vi "Test CVT.vi"() -> ()   [LabVIEW 2014, in "Controller.lvlib" / "Controller.lvclass"]
uses:
  Controller.lvclass
panel:
  out "data value":variant
  out "json cvt":string
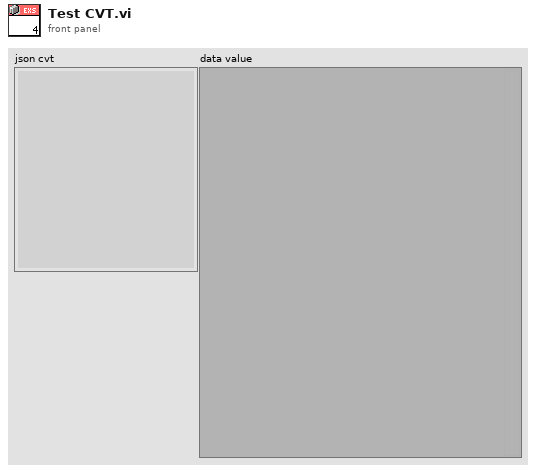
[diagram p1: front panel]
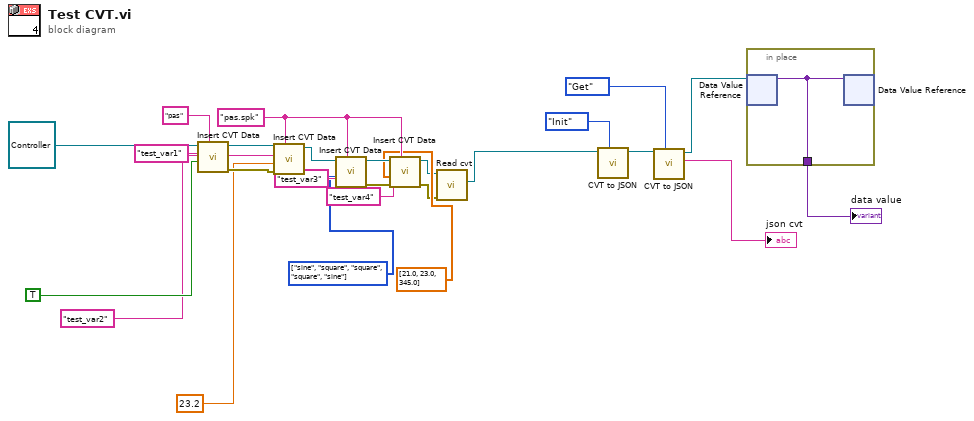
[diagram p0: block diagram]
diagram:
  w8 = enum16{"sine", "square"}[] [enum."sine", enum."square", enum."square", enum."square", enum."sine"] items=["sine", "square"]
  w5 = "pas.spk" ("Group")
  n1 = call "Insert CVT Data.vi"("Group"="pas", "Data"=TRUE, "tag"="test_var1", "Controller in"=refnum<class "Controller.lvclass"> refnum ("Controller.lvlib:Controller")) -> ("error out"=w20:errorcluster, "Controller out"=w21:refnum<class "Controller.lvclass">)  [unwired: 6 in]
  n2 = call "Insert CVT Data.vi"("Group"=w5, "error in"=w20, "Data"=23.2, "tag"="test_var2", "Controller in"=w21) -> ("Controller out"=w10:refnum<class "Controller.lvclass">)  [unwired: 5 in, 1 out]
  n3 = call "Insert CVT Data.vi"("Group"=w5, "Data"=w8, "tag"="test_var3", "Controller in"=w10) -> ("error out"=w6:errorcluster, "Controller out"=w7:refnum<class "Controller.lvclass">)  [unwired: 6 in]
  n4 = call "Insert CVT Data.vi"("Group"=w5, "error in"=w6, "Data"=dbl[] [21.0, 23.0, 345.0], "tag"="test_var4", "Controller in"=w7) -> ("error out"=w1:errorcluster, "Controller out"=w2:refnum<class "Controller.lvclass">)  [unwired: 5 in]
  n5 = call "Read cvt.vi"("error in (no error)"=w1, "Controller in"=w2) -> ("cvt"=w17:refnum<data-value>)  [unwired: 7 in, 2 out]
  n6 = call "CVT to JSON.vi"("Select"=enum16{"Init", "Get", "Destroy"}."Init", "cvt in"=w17) -> ("cvt out"=w15:refnum<data-value>)  [unwired: 7 in, 2 out]
  n7 = call "CVT to JSON.vi"("Select"=enum16{"Init", "Get", "Destroy"}."Get", "cvt in"=w15) -> ("json cvt"=→"json cvt":string, "cvt out"=w12:refnum<data-value>)  [unwired: 7 in, 1 out]
  n8 = in-place {
    in-place-border: [w26] -> w11
    n9 = in-place-dvr #1(w12) -> (w26:variant)  [unwired: 1 out]
    n10 = in-place-dvr #1(w26) -> ()  [unwired: 2 out]
  }
  "data value" <- w11
